vi "Do.vi"(8 "error in":errorcluster, 10 "Actor in":refnum<class "Actor.lvclass">, 11 "Get Device Data MSG":refnum<class "Get Device Data MSG.lvclass">) -> (0 "error out":errorcluster, 2 "Actor out":refnum<class "Actor.lvclass">)   [LabVIEW 2014, in "DAQ Device.lvlib" / "Get Device Data MSG.lvclass"]
doc: "(<B>Filename</B>: Actor Framework.lvlib:Message.lvclass:Do.vi)\n\nDefines what a message does when it is received by an actor. Generally, a message instructs an actor to invoke one of its methods. By default, this method does nothing. A child class must override it to define behavior. Create a child class by using the Actor Framework Message Maker dialog box."
uses:
  Get Device Data MSG.lvclass
  <vilib>/ActorFramework/Actor/Actor.lvclass
  Device.lvclass
  Device.lvclass/Device.ctl
  Messages/Send Data Msg.lvclass/Send Data Msg.ctl
  Read Configurable Device.vi
  Read Send Data MSG.vi
  Messages/Write Data.vi
  Devices/Configurable Device/Configurable Device.lvclass
  Messages/Send Data Msg.lvclass
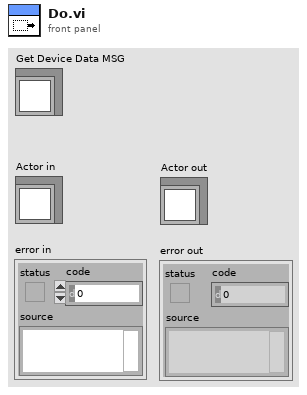
[diagram p1: front panel]
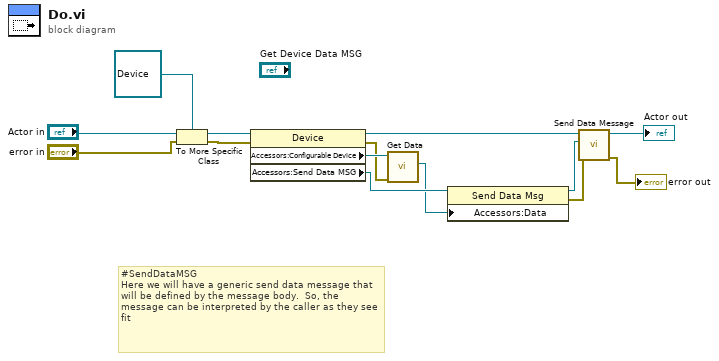
[diagram p0: block diagram]
diagram:
  # "#SendDataMSG\nHere we will have a generic send data message that will be defined by the message body.  So, the message can be interpreted by the caller as they see fit"
  n1 = To More Specific Class(target class=refnum<class "Device.lvclass"> refnum ("DAQ Device.lvlib:Device"), reference="Actor in", error in="error in") -> (specific class reference=w10:refnum<class "Device.lvclass">, error out=w11:errorcluster)
  n2 = property class="Device"(reference=w10, error in=w11) -> (reference out=w7:refnum<class "Device.lvclass">, error out=w8:errorcluster, "Accessors:Configurable Device"=w9:refnum<class "Configurable Device.lvclass">, "Accessors:Send Data MSG"=w4:refnum<class "Send Data Msg.lvclass">)
  n3 = call-dynamic "Get Data.vi"("error in (no error)"=w8, "Configurable Device in"=w9) -> ("DataOut"=w3:refnum<class "Data.lvclass">)  [unwired: 7 in, 2 out]
  n4 = property class="Send Data Msg"(reference=w4, "Accessors:Data"=w3) -> (reference out=w2:refnum<class "Send Data Msg.lvclass">, error out=w1:errorcluster)  [unwired: 1 in]
  n5 = call "Send Data Message.vi"("error in"=w1, "SendDataMSG"=w2, "Device in"=w7) -> ("error out"=→"error out":errorcluster, "Device out"=→"Actor out":refnum<class "Device.lvclass">)  [unwired: 7 in]
